vi "UDP Vision - Sender.vi"(9 "local port":u16=1180, 11 "Image":T1(plugin-control)) -> ()   [LabVIEW 2023]
doc: "The UDP protocol differs from TCP in that there is no error-checking with the packets of information that are sent, and thus no guarantee whatsoever that an intended recipient will actually receive a given piece of data.\n\nUDP does offer the ability to \"broadcast\" data across a network--simply specify an IP Address of all ones (255.255.255.255) to attempt to broadcast information network-wide. Keep in mind that routers and other network hardware will generally refuse to forward the broadcast beyond certain points, so the extent of the broadcast will in practice be limited."
uses:
  UDP Main States.ctl
panel:
  out "Driver Station address":string
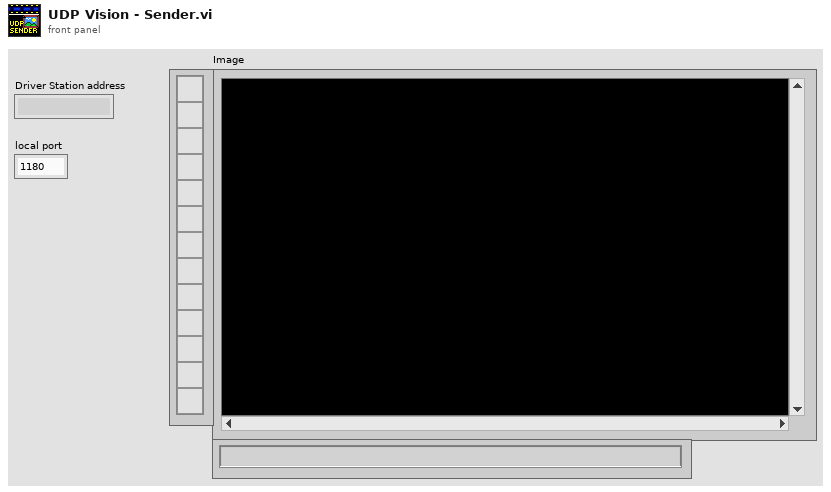
[diagram p1: front panel]
types:
  T1 = typedef "IMAQ Image.ctl" = refnum<image>
  T2 = typedef "UDP Main States.ctl" = enum16{"Message Dispatcher", "INI", "Send Data", "UDP Close", "UDP Open", "Exit"}
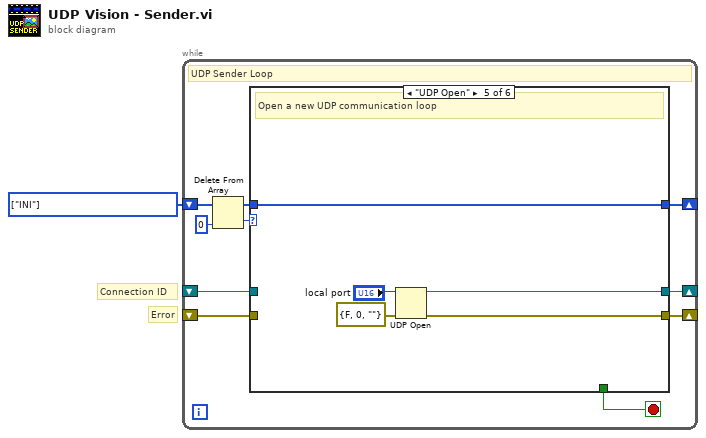
[diagram p0: block diagram]
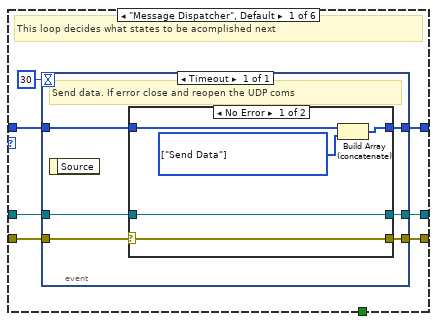
[diagram p2: hidden frame]
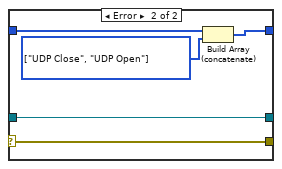
[diagram p3: hidden frame]
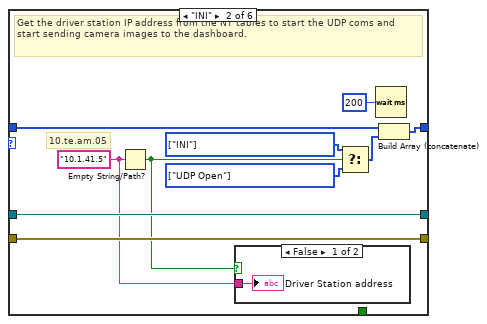
[diagram p4: hidden frame]
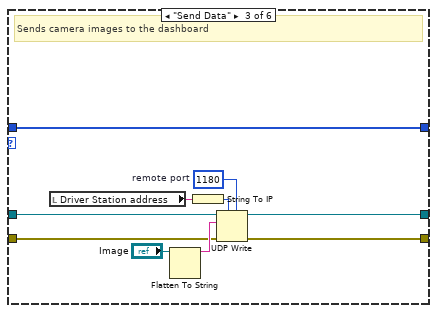
[diagram p6: hidden frame]
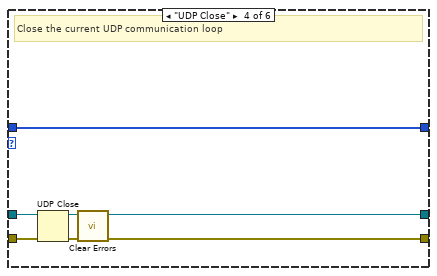
[diagram p7: hidden frame]
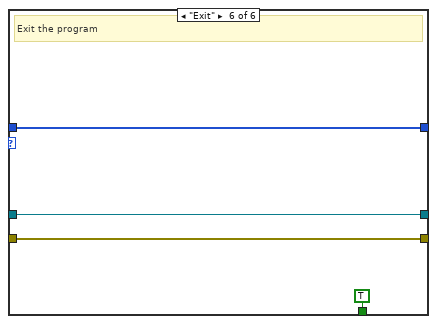
[diagram p8: hidden frame]
diagram:
  w1 = T2[] [enum."INI"] items=["Message Dispatcher", "INI", "Send Data", "UDP Close", "UDP Open", "Exit"]
  # "Error"
  # "Connection ID"
  n1 = while {
    shift-right: [w3] -> _
    shift-left: w1 -> [w7]
    shift-right: [w11] -> _
    shift-left: _ -> [w9]
    shift-right: [w10] -> _
    shift-left: _ -> [w8]
    stop <- w2 stop-if-true
    # "UDP Sender Loop"
    n2 = Delete From Array(array=w7, index=0) -> (deleted portion=w5:T2, array with subset deleted=w4:T2[])  [unwired: 1 in]
    n3 = case shown="\"UDP Open\"" w5 {
      tunnel: [w15 w44 w51 w56 w65 w70] -> w11
      tunnel: [w13 w43 w50 w57 w64 w69] -> w10
      tunnel: w9 -> [w16 w44 w53 w60 _ w70]
      tunnel: w8 -> [w14 w43 w52 w59 _ w69]
      tunnel: w4 -> [w18 w42 w49 w61 w62 w68]
      tunnel: [w17 w40 w49 w61 w62 w68] -> w3
      tunnel: [_ _ _ _ _ TRUE] -> w2
      frame "Message Dispatcher", Default {
        # "This loop decides what states to be acomplished next"
        n4 = event shown="[0] Timeout" {
          selector: _ -> [_]
          dyn-events: _ -> [_]
          timeout: 30 -> [_]
          tunnel: w18 -> [w22]
          tunnel: [w21] -> w17
          tunnel: w16 -> [w20]
          tunnel: [w19] -> w15
          tunnel: w14 -> [w24]
          tunnel: [w23] -> w13
          event Timeout {
            # "Send data. If error close and reopen the UDP coms"
            n5 = event-data() -> ()  [unwired: 1 in, 1 out]
            n6 = case shown="No Error" w24 {
              selector: w24 -> [w29 w34]
              tunnel: [w29 w34] -> w23
              tunnel: w22 -> [w28 w33]
              tunnel: [w26 w31] -> w21
              tunnel: w20 -> [w27 w32]
              tunnel: [w27 w32] -> w19
              frame No Error {
                w25 = T2[] [enum."Send Data"] items=["Message Dispatcher", "INI", "Send Data", "UDP Close", "UDP Open", "Exit"]
                n7 = Build Array (concatenate)(w28, w25) -> (w26:T2[])
              }
              frame Error {
                w30 = T2[] [enum."UDP Close", enum."UDP Open"] items=["Message Dispatcher", "INI", "Send Data", "UDP Close", "UDP Open", "Exit"]
                n8 = Build Array (concatenate)(w33, w30) -> (w31:T2[])
              }
            }
          }
        }
      }
      frame "INI" {
        w35 = "10.1.41.5"
        w38 = T2[] [enum."INI"] items=["Message Dispatcher", "INI", "Send Data", "UDP Close", "UDP Open", "Exit"]
        w39 = T2[] [enum."UDP Open"] items=["Message Dispatcher", "INI", "Send Data", "UDP Close", "UDP Open", "Exit"]
        # "10.te.am.05"
        # "Get the driver station IP address from the NT tables to start the UDP coms and start sending camera images to the dashboard."
        n9 = Empty String/Path?(string/path=w35) -> (empty?=w36:bool)
        n10 = case shown="False" w36 {
          tunnel: w35 -> [w45 _]
          frame False {
            "Driver Station address" <- w45
          }
          frame True {
          }
        }
        n11 = Select(t=w38, s=w36, f=w39) -> (s? t:f=w37:T2[])
        n12 = Wait (ms)(milliseconds to wait=u32 200) -> ()  [unwired: 1 out]
        n13 = Build Array (concatenate)(w42, w37) -> (w40:T2[])
      }
      frame "Send Data" {
        w47 = u16 1180  # remote port
        # "Sends camera images to the dashboard"
        n14 = local read "Driver Station address"() -> (w46:string)
        n15 = Flatten To String(anything="Image") -> (data string=w55:string)  [unwired: 3 in, 2 out]
        n16 = String To IP(1:w46) -> (0:w48:u32)
        n17 = UDP Write(address=w48, port or service name=w47, connection ID=w53, data in=w55, 8:w52) -> (error out=w50:errorcluster, 3:w51:refnum<k16>)  [unwired: 1 in]
      }
      frame "UDP Close" {
        # "Close the current UDP communication loop"
        n18 = UDP Close(connection ID=w60, 8:w59) -> (connection ID out=w56:refnum<k16>, error out=w58:errorcluster)
        n19 = call <vilib>:"Clear Errors.vi"("error in (no error)"=w58) -> ("error out"=w57:errorcluster)  [unwired: 5 in, 1 out]
      }
      frame "UDP Open" {
        # "Open a new UDP communication loop"
        n20 = UDP Open(8:errorcluster {"status"=FALSE, "code"=0, "source"=""} ("error in (no error)"), 11:"local port") -> (port=w65:refnum<k16>, 0:w64:errorcluster)  [unwired: 3 in, 1 out]
      }
      frame "Exit" {
        # "Exit the program"
      }
    }
  }
